vi "layout.vi"(0 "reference in":refnum<class "DQMHModuleNode.lvclass">, 1 "graph":refnum<class "Graph.lvclass">, 2 "graphics":refnum<class "Graphics.lvclass">, 3 "grid":refnum<class "Grid.lvclass">, 5 "error in (no error)":errorcluster) -> (14 "reference out":refnum<class "DQMHModuleNode.lvclass">, 19 "error out":errorcluster)   [LabVIEW 2014, in "DQMHModuleNode.lvclass"]
doc: "public void layout(Graph g, Graphics2D g2, Grid grid)"
uses:
  <resource>/Framework/Providers/Open_GDS/UML/DQMHModuleNode_class/DQMHModuleNode.lvclass
  <resource>/Framework/Providers/Open_GDS/UML/Graph_class/Graph.lvclass
  <resource>/Framework/Providers/Open_GDS/UML/Graphics_class/Graphics.lvclass
  <resource>/Framework/Providers/Open_GDS/UML/Grid_class/Grid.lvclass
  <resource>/Framework/Providers/Open_GDS/UML/General/Rectangle/Rectangle Rectangle2D.ctl
  <resource>/Framework/Providers/Open_GDS/UML/MultiLineString_class/MultiLineString.lvclass
  <resource>/Framework/Providers/Open_GDS/UML/RectangularNode_class/RectangularNode.lvclass
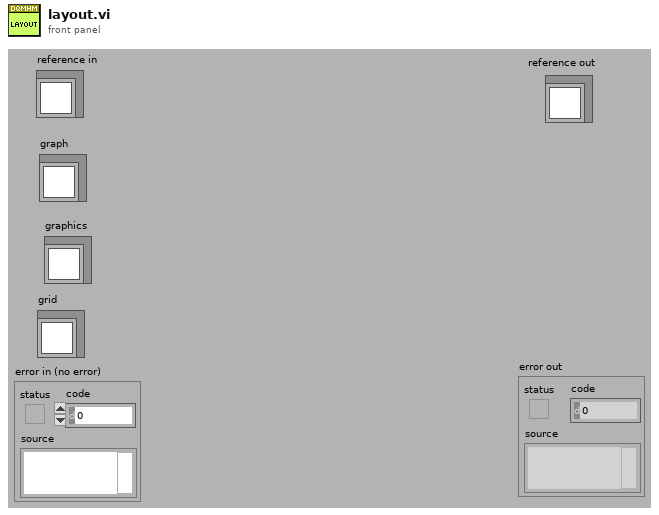
[diagram p1: front panel]
types:
  T1 = typedef "Rectangle Rectangle2D.ctl" = cluster{"x":dbl, "y":dbl, "width":dbl, "height":dbl}
  T2 = typedef "DQMHModuleNode.lvclass/ObjectAttributes.ctl" = cluster{"midHeight":dbl, "botHeight":dbl, "Name":refnum<class "MultiLineString.lvclass">, "Description":refnum<class "MultiLineString.lvclass">, "InternalData":refnum<class "MultiLineString.lvclass">, "Events":refnum<class "MultiLineString.lvclass">, "DEFAULT_COMPARTMENT_HEIGHT":i32, "DEFAULT_WIDTH":i32, "DEFAULT_HEIGHT":i32, "showEvents":bool, "showInternalData":bool, "ClassPath":path, "Template":string, "Icon":u8[][]}
  T3 = typedef "RectangularNode.lvclass/ObjectAttributes.ctl" = cluster{"bounds":T1}
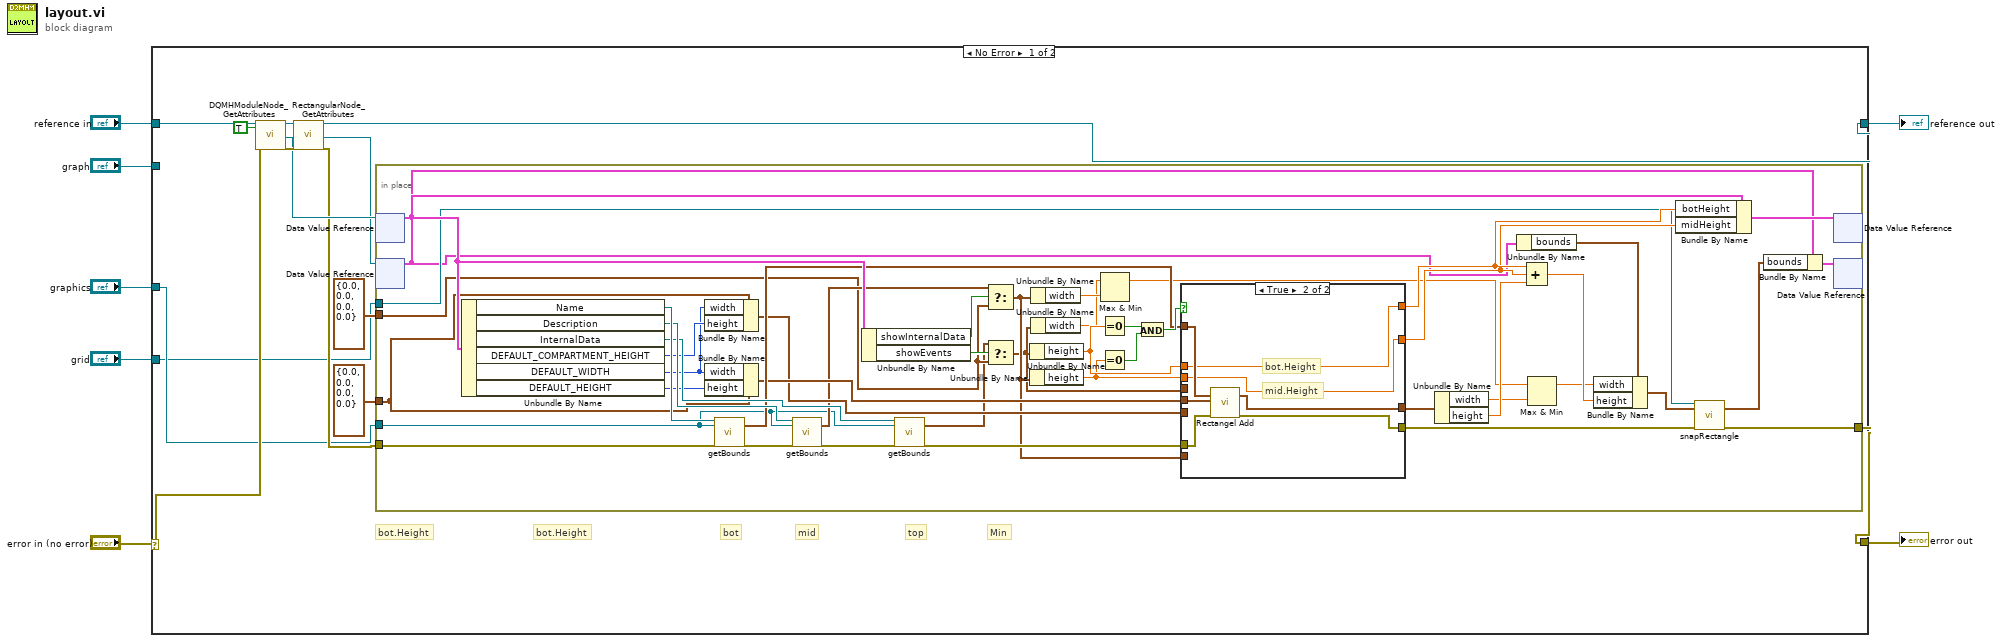
[diagram p0: block diagram]
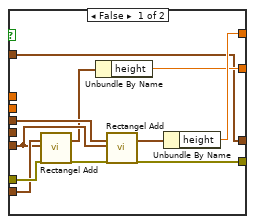
[diagram p2: hidden frame]
diagram:
  n1 = case shown="No Error" "error in (no error)" {
    selector: "error in (no error)" -> [w18 w87]
    tunnel: "reference in" -> [w21 w88]
    tunnel: [w20 w87] -> w6
    tunnel: [w19 w88] -> w5
    tunnel: "graph" -> [_ _]
    tunnel: "graphics" -> [w10 _]
    tunnel: "grid" -> [w8 _]
    frame No Error {
      # "mid.Height"
      # "bot.Height"
      # "mid.Height"
      # "bot.Height"
      # "bot"
      # "mid"
      # "top"
      # "Min"
      n2 = call <resource>:"DQMHModuleNode_GetAttributes.vi"("reference in"=w21, "OnlyGetDvrReference(False)"=TRUE, "error in (no error)"=w18) -> ("reference out"=w16:refnum<class "DQMHModuleNode.lvclass">, "DataRef"=w14:refnum<data-value>, "error out"=w15:errorcluster)  [unwired: 13 in, 1 out]
      n3 = call <resource>:"RectangularNode_GetAttributes.vi"("reference in"=w16, "error in (no error)"=w15) -> ("reference out"=w19:refnum<class "DQMHModuleNode.lvclass">, "DataRef"=w13:refnum<data-value>, "error out"=w11:errorcluster)  [unwired: 14 in, 1 out]
      n4 = in-place {
        in-place-border: T1 {"x"=0.0, "y"=0.0, "width"=0.0, "height"=0.0} ("f") -> [w42]
        in-place-border: w11 -> [w40]
        in-place-border: w10 -> [w37]
        in-place-border: T1 {"x"=0.0, "y"=0.0, "width"=0.0, "height"=0.0} ("bounds") -> [w36]
        in-place-border: w8 -> [w31]
        in-place-border: [w28] -> w20
        n5 = in-place-dvr #1(w14) -> (w68:T2)  [unwired: 1 out]
        n6 = in-place-dvr #2(w13) -> (w23:T3)  [unwired: 1 out]
        n7 = Unbundle By Name(w68) -> ("Name"=w62:refnum<class "MultiLineString.lvclass">, "Description"=w61:refnum<class "MultiLineString.lvclass">, "InternalData"=w60:refnum<class "MultiLineString.lvclass">, "DEFAULT_COMPARTMENT_HEIGHT"=w59:i32, "DEFAULT_WIDTH"=w58:i32, "DEFAULT_HEIGHT"=w57:i32)
        n8 = Bundle By Name(cluster=w36, "width"=w58, "height"=w59) -> (w52:T1)
        n9 = Bundle By Name(cluster=w36, "width"=w58, "height"=w57) -> (w54:T1)
        n10 = call-dynamic "getBounds.vi"("reference"=w62, "graphics"=w37, "error in (no error)"=w40) -> ("bounds"=w55:T1, "error out"=w39:errorcluster)  [unwired: 15 out]
        n11 = call-dynamic "getBounds.vi"("reference"=w61, "graphics"=w37, "error in (no error)"=w39) -> ("bounds"=w43:T1, "error out"=w38:errorcluster)  [unwired: 15 out]
        n12 = Unbundle By Name(w68) -> ("showInternalData"=w64:bool, "showEvents"=w63:bool)
        n13 = call-dynamic "getBounds.vi"("reference"=w60, "graphics"=w37, "error in (no error)"=w38) -> ("bounds"=w41:T1, "error out"=w53:errorcluster)  [unwired: 15 out]
        n14 = Select(t=w43, s=w64, f=w42) -> (s? t:f=w51:T1)
        n15 = Select(t=w41, s=w63, f=w42) -> (s? t:f=w50:T1)
        n16 = Unbundle By Name(w50) -> ("height"=w49:dbl)
        n17 = Unbundle By Name(w51) -> ("height"=w48:dbl)
        n18 = Unbundle By Name(w51) -> ("width"=w33:dbl)
        n19 = Unbundle By Name(w50) -> ("width"=w32:dbl)
        n20 = Equal To 0?(x=w49) -> (x = 0?=w34:bool)
        n21 = Equal To 0?(x=w48) -> (x = 0?=w35:bool)
        n22 = Max & Min(x=w32, y=w33) -> (max(x,y)=w24:dbl)  [unwired: 1 out]
        n23 = And(x=w34, y=w35) -> (x .and. y?=w56:bool)
        n24 = case shown="True" w56 {
          tunnel: w55 -> [w69 w86]
          tunnel: w54 -> [_ w85]
          tunnel: w53 -> [w79 w84]
          tunnel: w52 -> [w76 _]
          tunnel: w51 -> [w78 _]
          tunnel: w50 -> [w75 _]
          tunnel: w49 -> [_ w83]
          tunnel: [w72 w83] -> w67
          tunnel: w48 -> [_ w82]
          tunnel: [w71 w82] -> w66
          tunnel: [w70 w81] -> w47
          tunnel: [w69 w80] -> w46
          frame False {
            n25 = call <resource>:"Rectangel Add.vi"("bounds1"=w78, "bounds2"=w76, "error in (no error)"=w79) -> ("boundsAdded"=w74:T1, "error out"=w77:errorcluster)  [unwired: 2 in, 13 out]
            n26 = Unbundle By Name(w74) -> ("height"=w71:dbl)
            n27 = call <resource>:"Rectangel Add.vi"("bounds1"=w75, "bounds2"=w76, "error in (no error)"=w77) -> ("boundsAdded"=w73:T1, "error out"=w70:errorcluster)  [unwired: 2 in, 13 out]
            n28 = Unbundle By Name(w73) -> ("height"=w72:dbl)
          }
          frame True {
            # "mid.Height"
            # "bot.Height"
            n29 = call <resource>:"Rectangel Add.vi"("bounds1"=w86, "bounds2"=w85, "error in (no error)"=w84) -> ("boundsAdded"=w80:T1, "error out"=w81:errorcluster)  [unwired: 2 in, 13 out]
          }
        }
        n30 = Unbundle By Name(w46) -> ("width"=w27:dbl, "height"=w45:dbl)
        n31 = Unbundle By Name(w23) -> ("bounds"=w26:T1)
        n32 = Compound Arithmetic op=ADD(w67, w66, w45) -> (w44:dbl)
        n33 = Max & Min(x=w24, y=w27) -> (max(x,y)=w25:dbl)  [unwired: 1 out]
        n34 = Bundle By Name(cluster=w26, "width"=w25, "height"=w44) -> (w30:T1)
        n35 = Bundle By Name(cluster=w68, "botHeight"=w67, "midHeight"=w66) -> (w65:T2)
        n36 = call <resource>:"snapRectangle.vi"("reference"=w31, "bounds"=w30, "error in (no error)"=w47) -> ("boundsOut"=w29:T1, "error out"=w28:errorcluster)  [unwired: 15 out]
        n37 = Bundle By Name(cluster=w23, "bounds"=w29) -> (w22:T3)
        n38 = in-place-dvr #1(w65) -> ()  [unwired: 2 out]
        n39 = in-place-dvr #2(w22) -> ()  [unwired: 2 out]
      }
    }
    frame Error {
    }
  }
  "reference out" <- w5
  "error out" <- w6
